vi "Plot Legend NumRows.vi"(8 "error in (no error)":errorcluster, 11 "XY graph ref":refnum<vi>) -> (0 "error out":errorcluster, 3 "XY graph ref":refnum<vi>)   [LabVIEW 2021, in "RocketPlot.lvlib"]
uses:
  RocketPlot.lvlib
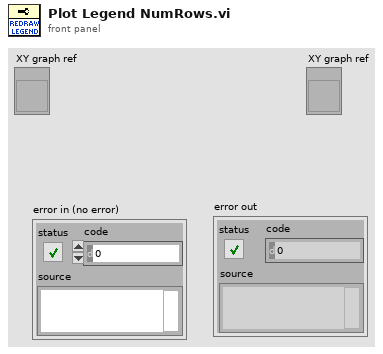
[diagram p1: front panel]
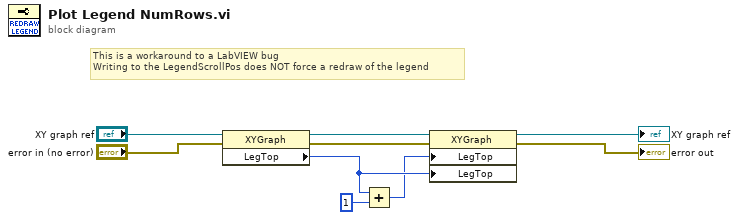
[diagram p0: block diagram]
diagram:
  # "This is a workaround to a LabVIEW bug\nWriting to the LegendScrollPos does NOT force a redraw of the legend"
  n1 = property class="XYGraph"(reference="XY graph ref", error in="error in (no error)") -> (reference out=w9:refnum<vi>, error out=w5:errorcluster, "LegTop"=w8:i32)
  n2 = Add(x=w8, y=1) -> (x+y=w6:i32)
  n3 = property class="XYGraph"(reference=w9, error in=w5, "LegTop"=w6, "LegTop"=w8) -> (reference out=→"XY graph ref":refnum<vi>, error out=→"error out":errorcluster)
